vi "Tosca-Initialize Indicators.vi"(0 "Input Events":T2[](array[typedef]), 5 "Digital Inputs":T1[](array[typedef]), 7 "DI Indicators":refnum<vi>, 9 "Event Indicators":refnum<vi>, 11 "error in (no error)":errorcluster) -> (15 "error out":errorcluster)   [LabVIEW 2020]
uses:
  Tosca-Input Event.ctl
  Tosca-Input Criterion.ctl
  epl-vi-lib/Utility VIs/Type Defs/Logic State.ctl
  Typedefs/Tosca-Accumulator.ctl
  Tosca-Digital Input.ctl
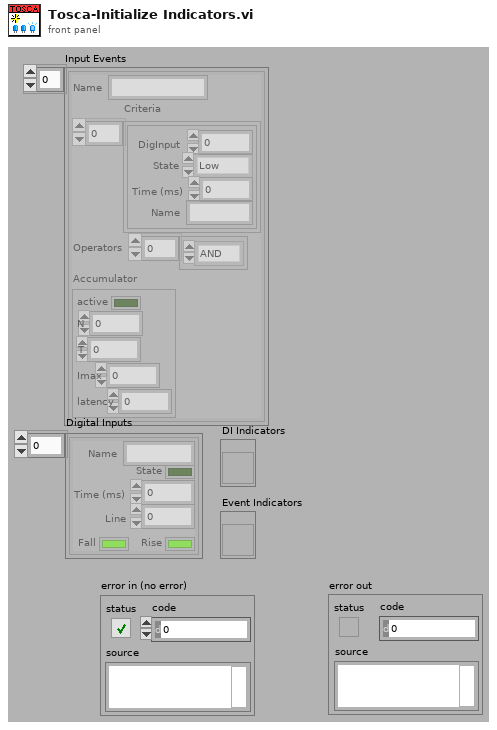
[diagram p1: front panel]
types:
  T1 = typedef "Tosca-Digital Input.ctl" = cluster{"Name":string, "State":bool, "Time (ms)":dbl, "Line":i32, "Rise":bool, "Fall":bool}
  T2 = typedef "Tosca-Input Event.ctl" = cluster{"Name":string, "Criteria":T3[], "Operators":enum16{"AND", "OR"}[], "Accumulator":T5}
  T3 = typedef "Tosca-Input Criterion.ctl" = cluster{"DigInput":i32, "State":T4, "Time (ms)":i32, "Name":string}
  T4 = typedef "Logic State.ctl" = enum16{"Low", "High", "Rising", "Falling"}
  T5 = typedef "Tosca-Accumulator.ctl" = cluster{"active":bool, "N":i32, "T":dbl, "Imax":dbl, "latency":dbl}
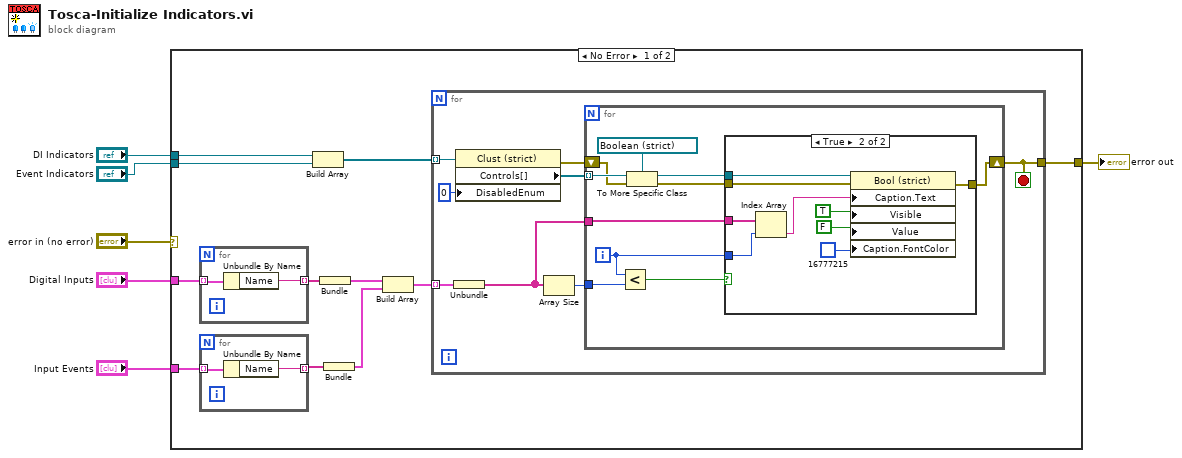
[diagram p0: block diagram]
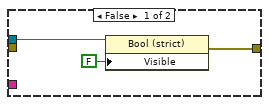
[diagram p2: hidden frame]
diagram:
  n1 = case shown="No Error" "error in (no error)" {
    selector: "error in (no error)" -> [_ w52]
    tunnel: "Digital Inputs" -> [w17 _]
    tunnel: "Input Events" -> [w16 _]
    tunnel: "DI Indicators" -> [w15 _]
    tunnel: "Event Indicators" -> [w12 _]
    tunnel: [w11 w52] -> w2
    frame No Error {
      n2 = for {
        tunnel: w17 -> [w51] mode=indexing
        tunnel: [w50] -> w14 mode=indexing
        n3 = Unbundle By Name(w51) -> ("Name"=w50:string)
      }
      n4 = for {
        tunnel: w16 -> [w49] mode=indexing
        tunnel: [w48] -> w9 mode=indexing
        n5 = Unbundle By Name(w49) -> ("Name"=w48:string)
      }
      n6 = Build Array(w15, w12) -> (w13:refnum<vi>[])
      n7 = Bundle(w14) -> (w10:cluster{string[]})  [unwired: 1 in]
      n8 = Bundle(w9) -> (w7:cluster{string[]})  [unwired: 1 in]
      n9 = Build Array(w10, w7) -> (w8:cluster{string[]}[])
      n10 = for {
        tunnel: w8 -> [w24] mode=indexing
        tunnel: w13 -> [w21] mode=indexing
        tunnel: [w20] -> w11
        stop <- w20 stop-if-true
        n11 = Unbundle(w24) -> (w19:string[])
        n12 = property class="Clust (strict)"(reference=w21, "DisabledEnum"=0) -> (error out=w22:errorcluster, "Controls[]"=w25:refnum<vi>[])  [unwired: 1 in, 1 out]
        n13 = Array Size(array=w19) -> (size(s)=w23:i32)
        n14 = for {
          tunnel: w25 -> [w34] mode=indexing
          tunnel: w19 -> [w31]
          tunnel: w23 -> [w33]
          shift-right: [w26] -> w20
          shift-left: w22 -> [w28]
          i -> [w30]
          n15 = Less?(x=w30, y=w33) -> (x < y?=w32:bool)
          n16 = To More Specific Class(target class=refnum<vi> refnum ("Boolean"), reference=w34, error in=w28) -> (specific class reference=w29:refnum<vi>, error out=w27:errorcluster)
          n17 = case shown="True" w32 {
            tunnel: w31 -> [_ w47]
            tunnel: w30 -> [_ w46]
            tunnel: w29 -> [w38 w43]
            tunnel: w27 -> [_ w41]
            tunnel: [w36 w40] -> w26
            frame False {
              n18 = property class="Bool (strict)"(reference=w38, "Visible"=FALSE) -> (error out=w36:errorcluster)  [unwired: 1 in, 1 out]
            }
            frame True {
              n19 = Index Array(array=w47, index=w46) -> (element=w42:string)
              n20 = property class="Bool (strict)"(reference=w43, error in=w41, "Caption.Text"=w42, "Visible"=TRUE, "Value"=FALSE, "Caption.FontColor"=u32 16777215) -> (error out=w40:errorcluster)  [unwired: 1 out]
            }
          }
        }
      }
    }
    frame Error {
    }
  }
  "error out" <- w2
